vi "Initialize.vi"(0 "Connection in":T1 {"Parity" items=["None", "Odd", "Even"]; "Flow Ctl" items=["None"]; "Baud" items=["4800"=4800, "9600"=9600, "19200"=19200, "38400"=38400]}, 3 "error in (no error)":errorcluster) -> (7 "Connection out":T1={"Baud"=9600, "Flow Ctl"=0, "COM port"="", "Parity"=0} {"Parity" items=["None", "Odd", "Even"]; "Flow Ctl" items=["None"]; "Baud" items=["4800"=4800, "9600"=9600, "19200"=19200, "38400"=38400]}, 8 "read buffer":string, 10 "error out":errorcluster)   [LabVIEW 2014, in "B&K Precision 9120 series.lvclass"]
uses:
  B&K Precision 9120 series.lvclass
  Serial_Config.ctl
  <vilib>/Instr/_visa.llb/VISA Set IO Buffer Mask.ctl
  <vilib>/Utility/error.llb/Error Cluster From Error Code.vi
  <vilib>/ErrorRing/Error Ring.xnode
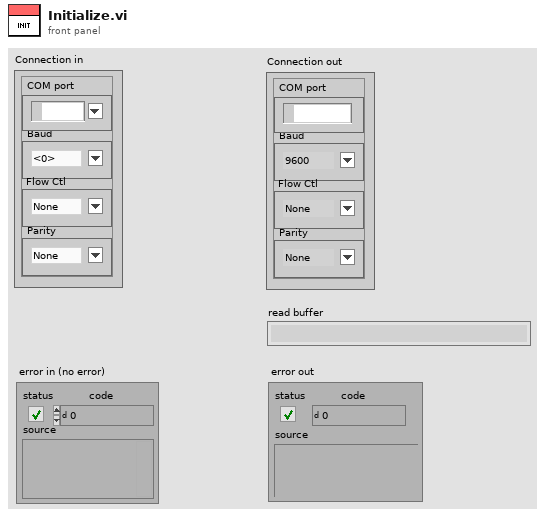
[diagram p1: front panel]
types:
  T1 = typedef "B&K Precision 9120 series.lvclass/Serial_Config.ctl" = cluster{"Baud":u32, "Flow Ctl":u16, "COM port":refnum<visa-resource-name>, "Parity":u16}
  T2 = typedef "VISA Set IO Buffer Mask.ctl" = u16
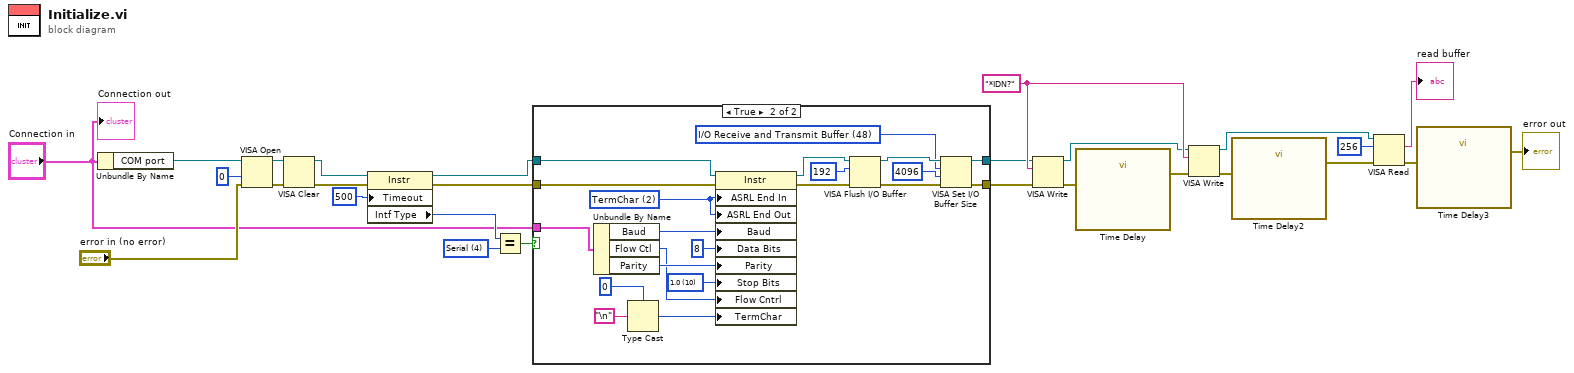
[diagram p0: block diagram]
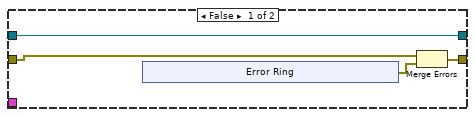
[diagram p2: hidden frame]
diagram:
  w13 = "*IDN?" ("write buffer")
  w19 = u16 4 items=["GPIB"=1, "VXI"=2, "GPIB-VXI"=3, "Serial"=4, "PXI"=5, "TCPIP"=6, "USB"=7] ("Interface Information:Interface Type")
  n1 = Unbundle By Name("Connection in") -> ("COM port"=w7:refnum<visa-resource-name>)
  n2 = VISA Open(access mode=0, error in (no error)="error in (no error)", VISA resource name=w7) -> (VISA resource name=w24:refnum<visa-resource-name>, error out=w25:errorcluster)  [unwired: 2 in]
  n3 = VISA Clear(VISA resource name=w24, error in (no error)=w25) -> (VISA resource name out=w23:refnum<visa-resource-name>, error out=w22:errorcluster)
  n4 = property class="Instr"(reference=w23, error in=w22, "Timeout"=u32 500 ("General Settings:Timeout Value")) -> (reference out=w17:refnum<visa-resource-name>, error out=w16:errorcluster, "Intf Type"=w20:u16)
  n5 = Equal?(x=w20, y=w19) -> (x = y?=w18:bool)
  n6 = case shown="True" w18 {
    tunnel: w17 -> [w31 w56]
    tunnel: w16 -> [w28 w55]
    tunnel: [w31 w38] -> w11
    tunnel: [w29 w37] -> w10
    tunnel: "Connection in" -> [_ w36]
    frame False {
      n7 = xnode "Error Ring"() -> ("error out"=w30:errorcluster)
      n8 = Merge Errors(w28, w30) -> (w29:errorcluster)
    }
    frame True {
      w40 = T2 48 items=["I/O Receive Buffer"=16, "I/O Transmit Buffer"=32, "I/O Receive and Transmit Buffer"=48] ("Mask")
      w46 = u16 2 items=["None", "Last Bit", "TermChar", "Break"] ("Serial Settings:End Mode for Writes")
      w52 = u16 10 items=["1.0"=10, "1.5"=15, "2.0"=20] ("Serial Settings:Stop Bits")
      n9 = Unbundle By Name(w36) -> ("Baud"=w47:u32, "Flow Ctl"=w51:u16, "Parity"=w53:u16)
      n10 = Type Cast(type=u8 0, x="\n") -> (*(type *) &x=w48:u8)
      n11 = property class="Instr"(reference=w56, error in=w55, "ASRL End In"=w46, "ASRL End Out"=w46, "Baud"=w47, "Data Bits"=u16 8 ("Serial Settings:Data Bits"), "Parity"=w53, "Stop Bits"=w52, "Flow Cntrl"=w51, "TermChar"=w48) -> (reference out=w45:refnum<visa-resource-name>, error out=w44:errorcluster)
      n12 = VISA Flush I/O Buffer(VISA resource name=w45, mask (16)=u16 192, error in (no error)=w44) -> (VISA resource name out=w42:refnum<visa-resource-name>, error out=w41:errorcluster)
      n13 = VISA Set I/O Buffer Size(VISA resource name=w42, mask (16)=w40, size (4096)=u32 4096, error in (no error)=w41) -> (VISA resource name out=w38:refnum<visa-resource-name>, error out=w37:errorcluster)
    }
  }
  n14 = VISA Write(VISA resource name=w11, write buffer=w13, error in (no error)=w10) -> (VISA resource name out=w12:refnum<visa-resource-name>, error out=w6:errorcluster)  [unwired: 1 out]
  n15 = call "Time Delay"("error in (no error)"=w6) -> ("error out"=w5:errorcluster)  [unwired: 10 in]
  n16 = VISA Write(VISA resource name=w12, write buffer=w13, error in (no error)=w5) -> (VISA resource name out=w14:refnum<visa-resource-name>, error out=w4:errorcluster)  [unwired: 1 out]
  n17 = call "Time Delay2"("error in (no error)"=w4) -> ("error out"=w3:errorcluster)  [unwired: 10 in]
  n18 = VISA Read(VISA resource name=w14, byte count=u32 256, error in (no error)=w3) -> (read buffer=→"read buffer":string, error out=w2:errorcluster)  [unwired: 2 out]
  n19 = call "Time Delay3"("error in (no error)"=w2) -> ("error out"=→"error out":errorcluster)  [unwired: 10 in]
  "Connection out" <- "Connection in"
